vi "Launch as Nested Actor.vi"(6 "timeout in ms (-1)":i32=-1, 8 "Error In":errorcluster, 9 "Panel":refnum<class "Panel.lvclass">, 10 "Panel Actor in":refnum<class "Panel Actor.lvclass">, 11 "Caller Actor in":refnum<class "Actor.lvclass">) -> (0 "Error Out":errorcluster, 2 "Actor's Enqueuer":refnum<class "Message Enqueuer.lvclass">, 3 "Caller Actor out":refnum<class "Actor.lvclass">)   [LabVIEW 2017, in "MGI-Panel Actor.lvlib" / "Panel Actor.lvclass"]
doc: "Launches a root panel as a nested actor of a non-panel actor.\n\n<B>Caller Actor In:</B> Nested caller Actor \n<B>Panel Actor In:</B> Panel actor to launch as nested actor\n<B>Panel:</B> Panel to use in displaying nested actor\n<B>timeout in ms</B> Time to wait for the panel to initialize\n<B>Error In:</B> Describes error conditions that occur before this node runs.\n\n<B>Caller Actor In:</B> Nested caller Actor \n<B>Actor's Enqueuer:</B> Enqueuer for newly spawned actor\n<B>Error Out:</B> Contains error information.\n----\nCopyright: MGI 2018\nAuthor: Derek Trepanier"
uses:
  Panel Actor.lvclass
  panel-manager/Source/Panel/Panel.lvclass
  <vilib>/ActorFramework/Message Enqueuer/Message Enqueuer.lvclass
  C:/Program Files (x86)/National Instruments/LabVIEW 2017/vi.lib/ActorFramework/Actor/Actor.lvclass
  <vilib>/ActorFramework/Actor/Actor.lvclass
  panel-manager/Source/Panel/Panel.lvclass/Panel.ctl
  Panel Actor.lvclass/Panel Actor.ctl
  panel-manager/Source/Init Waiter/Init Waiter.vi
  panel-manager/Source/Init Waiter/Init Waiter.lvclass
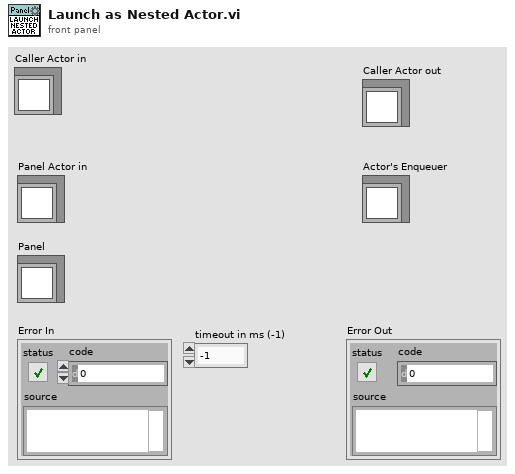
[diagram p1: front panel]
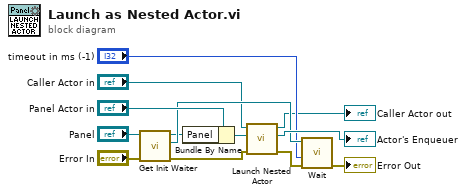
[diagram p0: block diagram]
diagram:
  n1 = call "Get Init Waiter.vi"("Error In"="Error In", "Panel In"="Panel") -> ("Error Out"=w8:errorcluster, "Init Waiter"=w7:refnum<class "Init Waiter.lvclass">, "Panel Out"=w1:refnum<class "Panel.lvclass">)  [unwired: 7 in]
  n2 = Bundle By Name(cluster="Panel Actor in", "Panel"=w1) -> (w12:refnum<class "Panel Actor.lvclass">)
  n3 = call <vilib>:"Launch Nested Actor.vi"("error in (no error)"=w8, "Nested Actor"=w12, "Caller Actor in"="Caller Actor in") -> ("error out"=w6:errorcluster, "Nested Actor's Enqueuer"=→"Actor's Enqueuer":refnum<class "Message Enqueuer.lvclass">, "Caller Actor out"=→"Caller Actor out":refnum<class "Actor.lvclass">)  [unwired: 6 in]
  n4 = call "Wait.vi"("Error In"=w6, "timeout in ms (-1)"="timeout in ms (-1)", "Init Waiter in"=w7) -> ("Error Out"=→"Error Out":errorcluster)  [unwired: 6 in, 2 out]
